vi "ProtocolAnswer.vi"(8 "error in":errorcluster caption="错误输入", 11 "IP":refnum<k5>) -> (0 "error out":errorcluster caption="错误输出", 1 "exit":bool, 3 "IP 2":refnum<k5>)   [LabVIEW 2014]
uses:
  <vilib>/Utility/error.llb/DialogType.ctl
  <vilib>/addons/database/Connection.llb/DB Tools Open Connec (String).vi
  <vilib>/addons/database/_DB Variant To Data/Database Variant To Data.xnode
  <vilib>/addons/database/NI_Database_API.lvlib
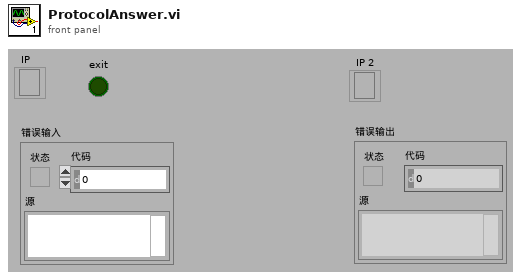
[diagram p1: front panel]
types:
  T1 = enum16{"open", "replace", "create", "open or create", "replace or create", "replace or create with confirmation"}
  T2 = typedef "DialogType.ctl" = u16
  T3 = typedef "NI_Database_API.lvlib/Conn ObjectReference.ctl" = refnum<k1>
  T4 = cluster{string, string, u8, string, u32, string}[]
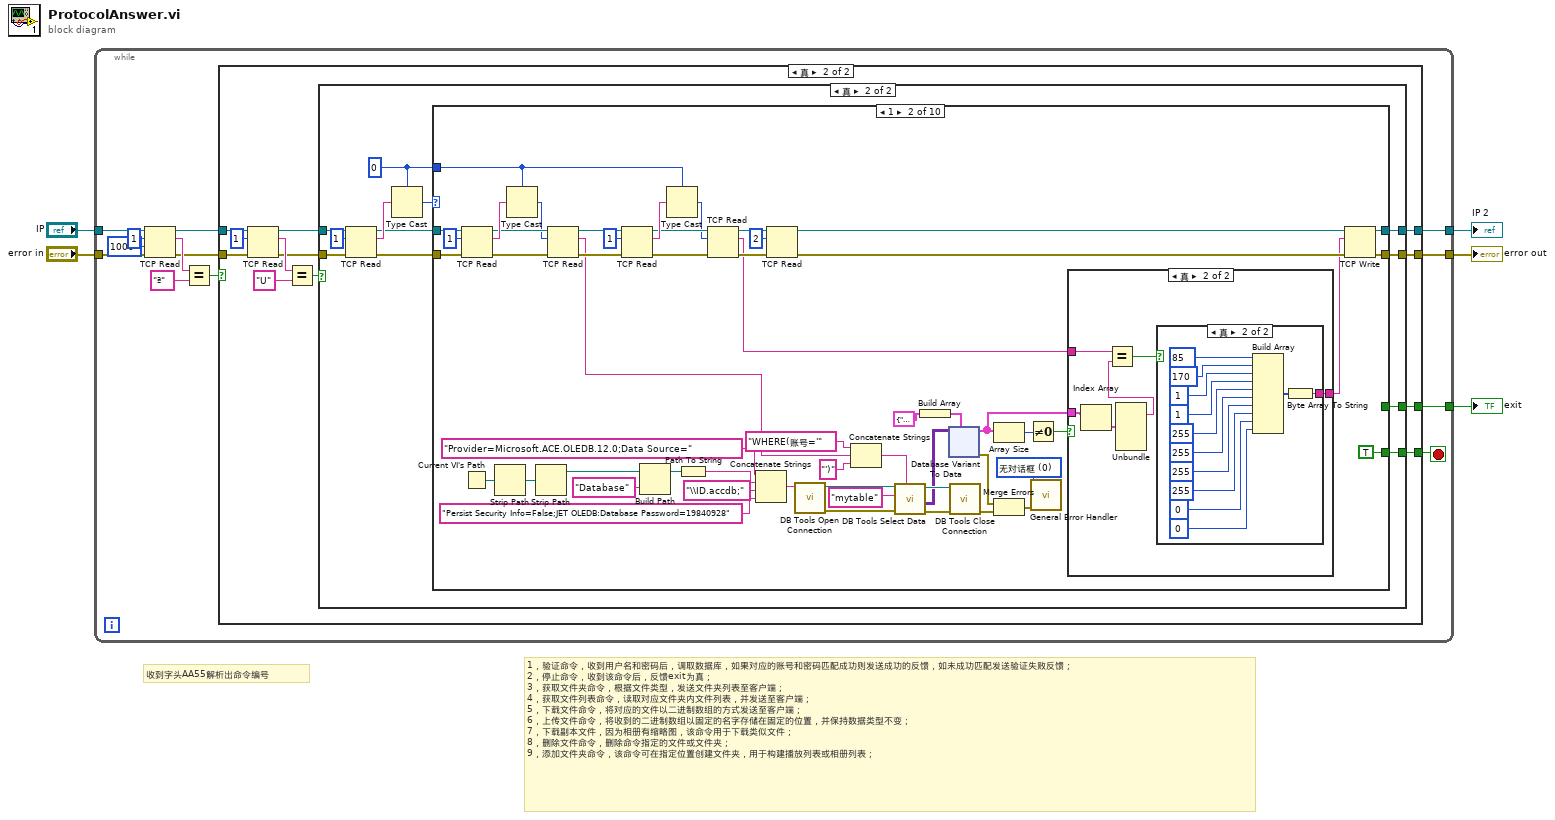
[diagram p0: block diagram]
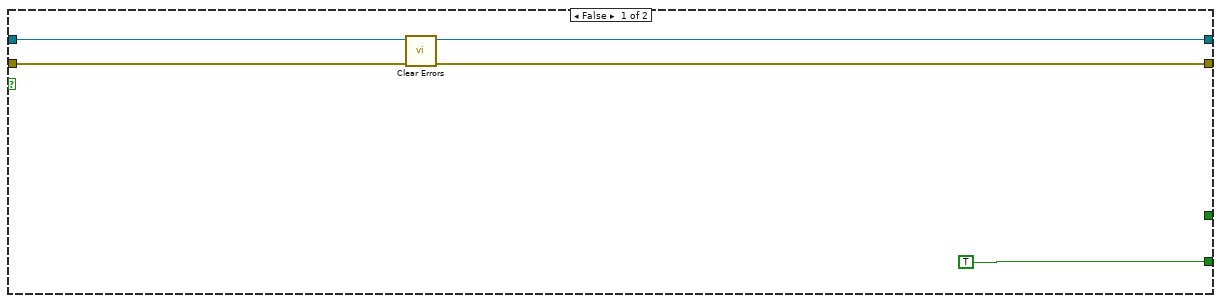
[diagram p2: hidden frame]
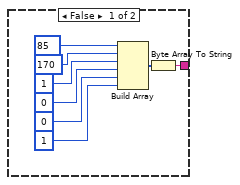
[diagram p5: hidden frame]
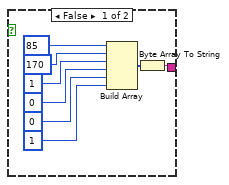
[diagram p6: hidden frame]
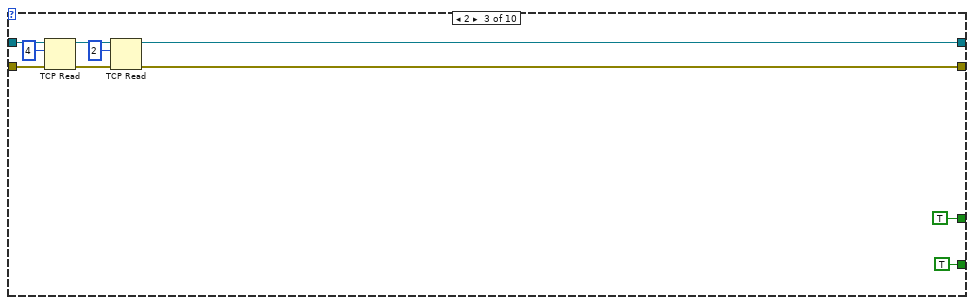
[diagram p7: hidden frame]
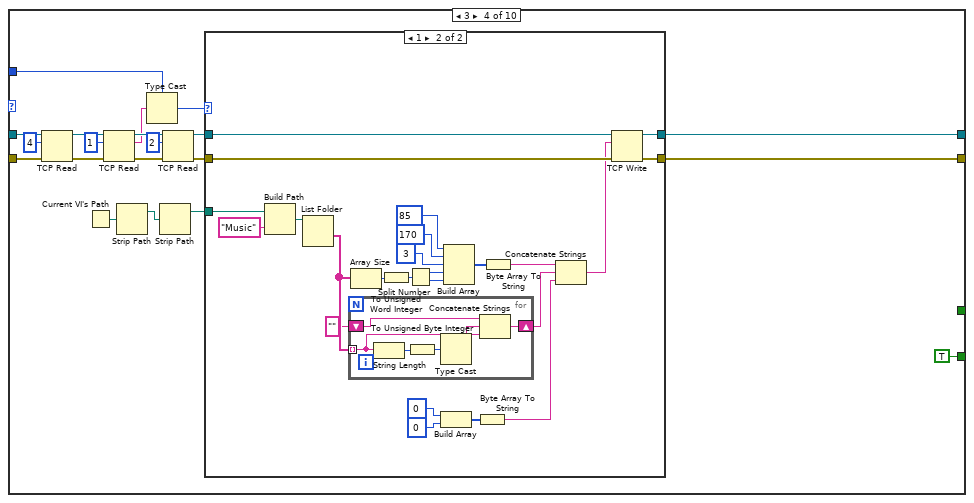
[diagram p8: hidden frame]
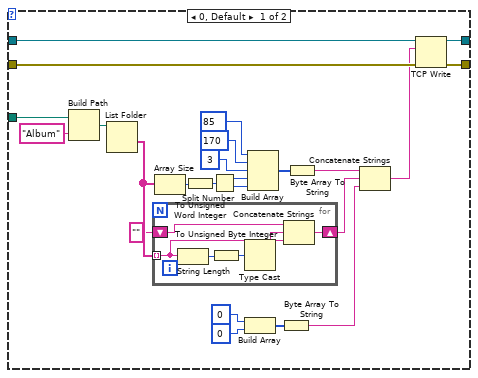
[diagram p9: hidden frame]
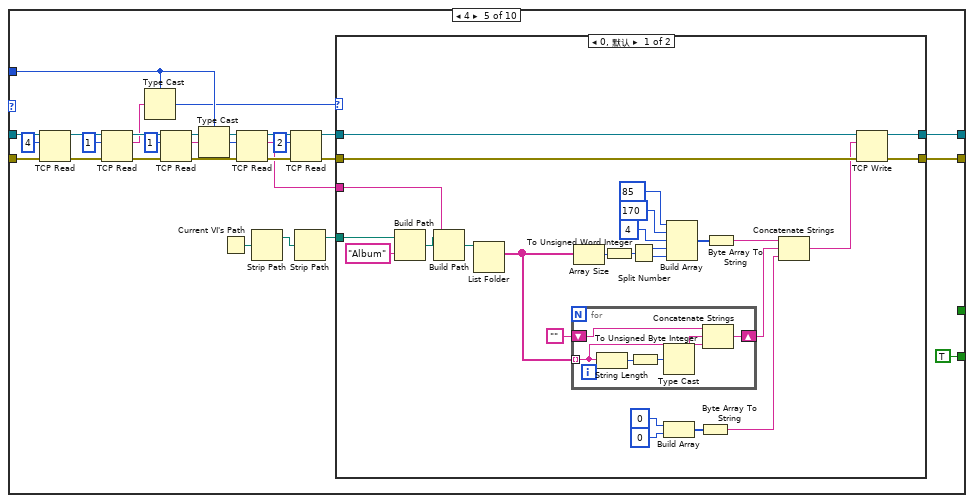
[diagram p10: hidden frame]
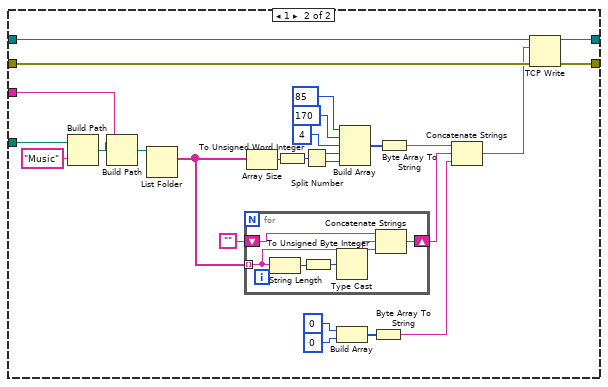
[diagram p11: hidden frame]
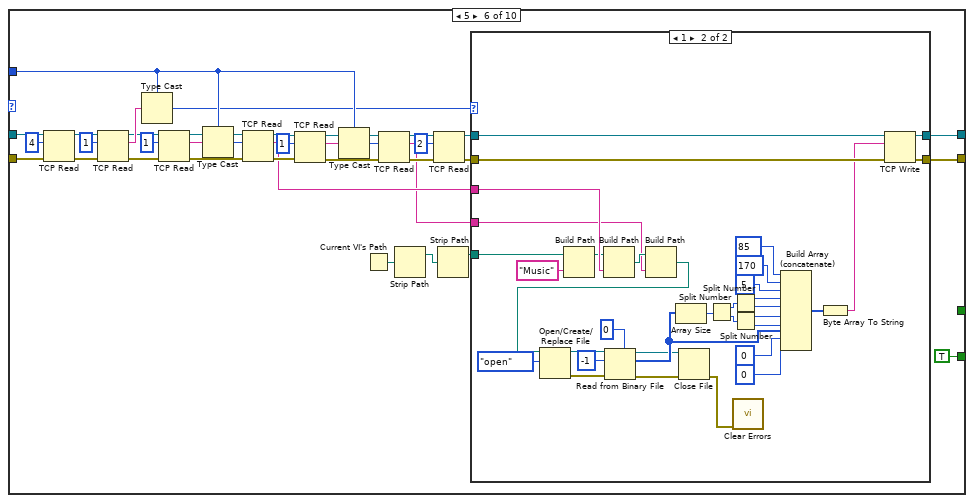
[diagram p12: hidden frame]
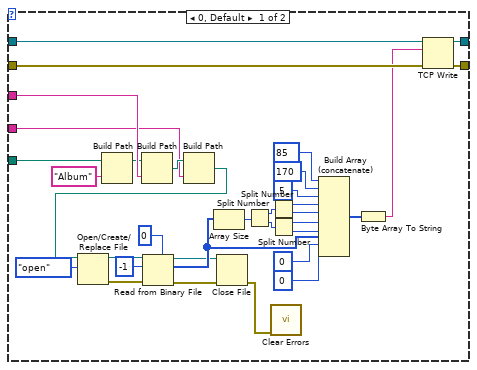
[diagram p13: hidden frame]
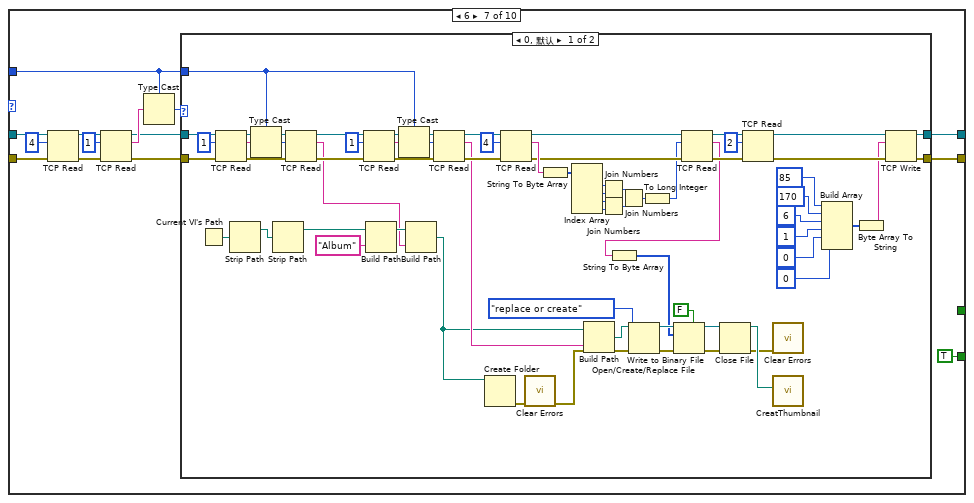
[diagram p14: hidden frame]
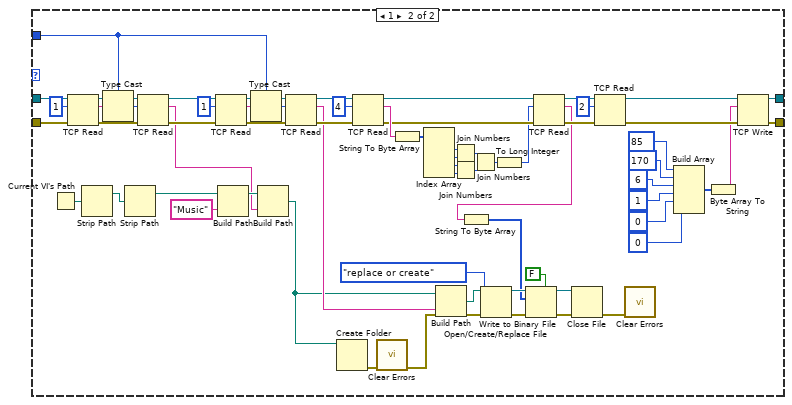
[diagram p15: hidden frame]
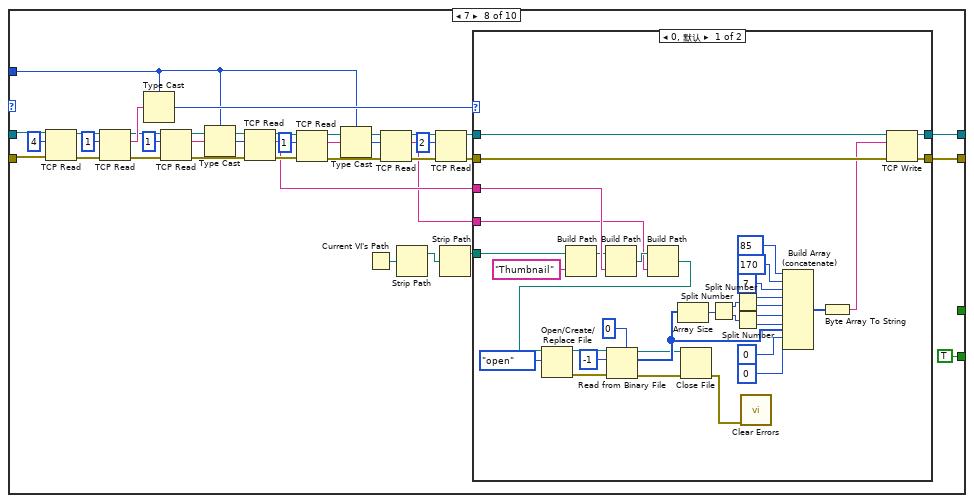
[diagram p16: hidden frame]
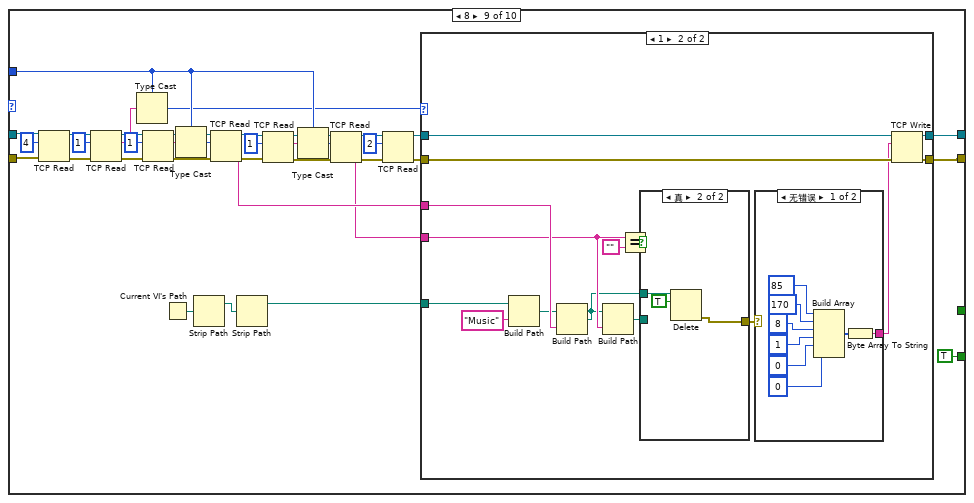
[diagram p18: hidden frame]
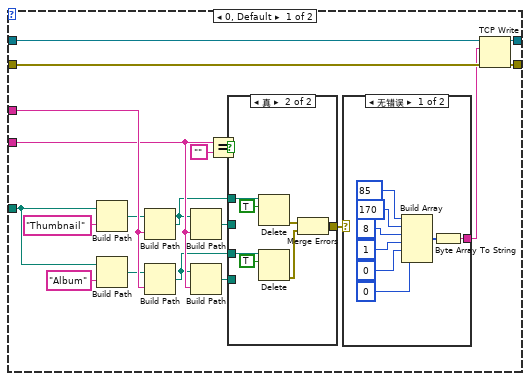
[diagram p19: hidden frame]
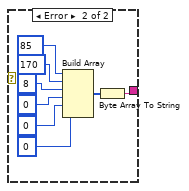
[diagram p20: hidden frame]
diagram:
  # "1，验证命令，收到用户名和密码后，调取数据库，如果对应的账号和密码匹配成功则发送成功的反馈，如未成功匹配发送验证失败反馈；\n2，停止命令，收到该命令后，反馈exit为真；\n3，获取文件夹命令，根据文件类型，发送文件夹列表至客户端；\n4，获取文件列表命令，读取对应文件夹内文件列表，并发送至客户端；\n5，下载文件命令，将对应的文件以二进制数组的方式发送至客户端；\n6，上传文件命令，将收到的二进制数组以固定的名字存储在固定的位置，并保持数据类型不变；\n7，下载副本文件，因为相册有缩略图，该命令用于下载类似文件；\n8，删除文件命令，删除命令指定的文件或文件夹；\n9，添加文件夹命令，该命令可在指定位置创建文件夹，用于构建播放列表或相册列表；"
  # "收到字头AA55解析出命令编号"
  n1 = while {
    tunnel: "IP" -> [w18]
    tunnel: "error in" -> [w17]
    tunnel: [w8] -> w3
    tunnel: [w7] -> w2
    tunnel: [w6] -> w1
    stop <- w9 stop-if-true
    n2 = TCP Read(connection ID=w18, bytes to read=1 ("读取的字节"), error in (no error)=w17, 9:1000 ("超时毫秒(25000)")) -> (connection ID out=w12:refnum<k5>, data out=w13:string, error out=w11:errorcluster)  [unwired: 1 in]
    n3 = Equal?(x=w13, y="ª") -> (x = y?=w10:bool)
    n4 = case shown="真" w10 {
      tunnel: w12 -> [w21 w33]
      tunnel: w11 -> [w20 w32]
      tunnel: [TRUE w26] -> w9
      tunnel: [w21 w25] -> w8
      tunnel: [w19 w24] -> w7
      tunnel: [_ w23] -> w6
      frame False {
        n5 = call <vilib>:"Clear Errors.vi"("error in (no error)"=w20) -> ("error out"=w19:errorcluster)  [unwired: 5 in, 1 out]
      }
      frame True {
        n6 = TCP Read(connection ID=w33, bytes to read=1 ("读取的字节"), error in (no error)=w32) -> (connection ID out=w28:refnum<k5>, data out=w31:string, error out=w27:errorcluster)  [unwired: 2 in]
        n7 = Equal?(x=w31, y="U") -> (x = y?=w29:bool)
        n8 = case shown="真" w29 {
          tunnel: w28 -> [w36 w48]
          tunnel: w27 -> [w35 w47]
          tunnel: [_ w41] -> w26
          tunnel: [w36 w39] -> w25
          tunnel: [w35 w38] -> w24
          tunnel: [_ w37] -> w23
          frame False {
          }
          frame True {
            w40 = u8 0
            n9 = TCP Read(connection ID=w48, bytes to read=1 ("读取的字节"), error in (no error)=w47) -> (connection ID out=w43:refnum<k5>, data out=w45:string, error out=w42:errorcluster)  [unwired: 2 in]
            n10 = Type Cast(type=w40, x=w45) -> (*(type *) &x=w44:u8)
            n11 = case shown="1" w44 {
              tunnel: w43 -> [w50 w102 w343 w363 w444 w551 w633 w770 w851 w970]
              tunnel: w42 -> [w49 w103 w340 w360 w443 w548 w631 w769 w850 w969]
              tunnel: [_ TRUE TRUE TRUE TRUE TRUE TRUE TRUE TRUE TRUE] -> w41
              tunnel: w40 -> [_ w89 _ w355 w440 w542 w621 w771 w849 w968]
              tunnel: [w50 w83 w339 w346 w426 w523 w622 w768 w845 w964] -> w39
              tunnel: [w49 w82 w336 w345 w425 w522 w623 w767 w844 w963] -> w38
              tunnel: [_ _ TRUE _ _ _ _ _ _ _] -> w37
              frame 0, Default {
              }
              frame 1 {
                w52 = T2 0 items=["无对话框", "确定信息", "继续或停止信息", "确定信息＋警告", "继续/停止+警告"] ("type of dialog (OK msg:1)")
                n12 = TCP Read(connection ID=w102, bytes to read=1 ("读取的字节"), error in (no error)=w103) -> (connection ID out=w99:refnum<k5>, data out=w100:string, error out=w98:errorcluster)  [unwired: 2 in]
                n13 = Current VI's Path() -> (path=w79:path)
                n14 = Strip Path(path=w79) -> (stripped path=w80:path)  [unwired: 1 out]
                n15 = Type Cast(type=w89, x=w100) -> (*(type *) &x=w97:u8)
                n16 = Strip Path(path=w80) -> (stripped path=w72:path)  [unwired: 1 out]
                n17 = TCP Read(connection ID=w99, bytes to read=w97, error in (no error)=w98) -> (connection ID out=w91:refnum<k5>, data out=w55:string, error out=w90:errorcluster)  [unwired: 2 in]
                n18 = TCP Read(connection ID=w91, bytes to read=1 ("读取的字节"), error in (no error)=w90) -> (connection ID out=w94:refnum<k5>, data out=w95:string, error out=w93:errorcluster)  [unwired: 2 in]
                n19 = Build Path(base path=w72, name or relative path="Database" ("名称或相对路径")) -> (appended path=w73:path)
                n20 = Type Cast(type=w89, x=w95) -> (*(type *) &x=w92:u8)
                n21 = Path To String(path=w73) -> (string=w63:string)
                n22 = TCP Read(connection ID=w94, bytes to read=w92, error in (no error)=w93) -> (connection ID out=w88:refnum<k5>, data out=w51:string, error out=w87:errorcluster)  [unwired: 2 in]
                n23 = Concatenate Strings("Provider=Microsoft.ACE.OLEDB.12.0;Data Source=", w63, "\\ID.accdb;", "Persist Security Info=False;JET OLEDB:Database Password=19840928" ("字符串")) -> (w65:string)
                n24 = TCP Read(connection ID=w88, bytes to read=2 ("读取的字节"), error in (no error)=w87) -> (connection ID out=w85:refnum<k5>, error out=w84:errorcluster)  [unwired: 2 in, 1 out]
                n25 = call-poly <vilib>:"DB Tools Open Connection.vi"("connection information"=w65) -> ("error out"=w67:errorcluster, "connection reference"=w66:T3)  [unwired: 7 in]
                n26 = Concatenate Strings("WHERE(账号='" ("condition"), w55, "')") -> (w77:string)
                n27 = call <vilib>:"DB Tools Select Data.vi"("condition"=w77, "error in (no error)"=w67, "table"="mytable", "connection reference"=w66) -> ("error out"=w70:errorcluster, "data"=w60:variant[][], "connection reference out"=w69:T3)  [unwired: 2 in]
                n28 = Build Array(cluster{string, string, u8, string, u32, string} {"", "", 0, "", 0, ""}) -> (w58:T4)
                n29 = xnode "Database Variant To Data"("database variant"=w60, "type"=w58) -> ("data"=w53:T4, "error out"=w56:errorcluster)  [unwired: 1 in]
                n30 = call <vilib>:"DB Tools Close Connection.vi"("error in (no error)"=w70, "connection reference"=w69) -> ("error out"=w61:errorcluster)  [unwired: 5 in]
                n31 = Array Size(array=w53) -> (size(s)=w78:i32)
                n32 = Merge Errors(w56, w61) -> (w57:errorcluster)
                n33 = Not Equal To 0?(x=w78) -> (x != 0?=w54:bool)
                n34 = call <vilib>:"General Error Handler.vi"("type of dialog (OK msg:1)"=w52, "error in (no error)"=w57) -> ()  [unwired: 9 in, 5 out]
                n35 = case shown="真" w54 {
                  tunnel: [w105 w118] -> w81
                  tunnel: w53 -> [_ w116]
                  tunnel: w51 -> [_ w115]
                  frame False {
                    n36 = Build Array(u8 85, u8 170, u8 1, u8 0, u8 0, u8 1) -> (w106:u8[])
                    n37 = Byte Array To String(unsigned byte array=w106) -> (string=w105:string)
                  }
                  frame True {
                    n38 = Index Array(array=w116) -> (element=w117:cluster{string, string, u8, string, u32, string})  [unwired: 1 in]
                    n39 = Unbundle(w117) -> (w114:string)  [unwired: 5 out]
                    n40 = Equal?(x=w115, y=w114) -> (x = y?=w113:bool)
                    n41 = case shown="真" w113 {
                      tunnel: [w119 w127] -> w118
                      frame False {
                        n42 = Build Array(u8 85, u8 170, u8 1, u8 0, u8 0, u8 1) -> (w120:u8[])
                        n43 = Byte Array To String(unsigned byte array=w120) -> (string=w119:string)
                      }
                      frame True {
                        n44 = Build Array(u8 85, u8 170, u8 1, u8 1, u8 255, u8 255, u8 255, u8 255, u8 0, u8 0) -> (w128:u8[])
                        n45 = Byte Array To String(unsigned byte array=w128) -> (string=w127:string)
                      }
                    }
                  }
                }
                n46 = TCP Write(connection ID=w85, data in=w81, error in (no error)=w84) -> (connection ID out=w83:refnum<k5>, error out=w82:errorcluster)  [unwired: 1 in, 1 out]
              }
              frame 2 {
                n47 = TCP Read(connection ID=w343, bytes to read=4 ("读取的字节"), error in (no error)=w340) -> (connection ID out=w342:refnum<k5>, error out=w337:errorcluster)  [unwired: 2 in, 1 out]
                n48 = TCP Read(connection ID=w342, bytes to read=2 ("读取的字节"), error in (no error)=w337) -> (connection ID out=w339:refnum<k5>, error out=w336:errorcluster)  [unwired: 2 in, 1 out]
              }
              frame 3 {
                n49 = TCP Read(connection ID=w363, bytes to read=4 ("读取的字节"), error in (no error)=w360) -> (connection ID out=w362:refnum<k5>, error out=w357:errorcluster)  [unwired: 2 in, 1 out]
                n50 = Current VI's Path() -> (path=w351:path)
                n51 = TCP Read(connection ID=w362, bytes to read=1 ("读取的字节"), error in (no error)=w357) -> (connection ID out=w359:refnum<k5>, data out=w356:string, error out=w354:errorcluster)  [unwired: 2 in]
                n52 = Strip Path(path=w351) -> (stripped path=w350:path)  [unwired: 1 out]
                n53 = Type Cast(type=w355, x=w356) -> (*(type *) &x=w352:u8)
                n54 = Strip Path(path=w350) -> (stripped path=w349:path)  [unwired: 1 out]
                n55 = TCP Read(connection ID=w359, bytes to read=2 ("读取的字节"), error in (no error)=w354) -> (connection ID out=w348:refnum<k5>, error out=w347:errorcluster)  [unwired: 2 in, 1 out]
                n56 = case shown="1" w352 {
                  tunnel: w349 -> [w388 w418]
                  tunnel: w348 -> [w376 w406]
                  tunnel: w347 -> [w374 w404]
                  tunnel: [w375 w405] -> w346
                  tunnel: [w373 w403] -> w345
                  frame 0, Default {
                    n57 = Build Path(base path=w388, name or relative path="Album" ("名称或相对路径")) -> (appended path=w386:path)
                    n58 = List Folder(path=w386) -> (folder names=w383:string[])  [unwired: 3 in, 3 out]
                    n59 = for {
                      tunnel: w383 -> [w390] mode=indexing
                      shift-right: [w392] -> w367
                      shift-left: "" -> [w389]
                      n60 = String Length(string=w390) -> (length=w394:i32)
                      n61 = To Unsigned Byte Integer(number=w394) -> (unsigned 8bit integer=w393:u8)
                      n62 = Type Cast(x=w393) -> (*(type *) &x=w391:string)  [unwired: 1 in]
                      n63 = Concatenate Strings(w389, w391, w390) -> (w392:string)
                    }
                    n64 = Array Size(array=w383) -> (size(s)=w385:i32)
                    n65 = To Unsigned Word Integer(number=w385) -> (unsigned 16bit integer=w384:u16)
                    n66 = Split Number(x=w384) -> (hi(x)=w381:u8, lo(x)=w380:u8)
                    n67 = Build Array(u8 0, u8 0) -> (w369:u8[])
                    n68 = Build Array(u8 85, u8 170, u8 3, w381, w380) -> (w372:u8[])
                    n69 = Byte Array To String(unsigned byte array=w369) -> (string=w366:string)
                    n70 = Byte Array To String(unsigned byte array=w372) -> (string=w368:string)
                    n71 = Concatenate Strings(w368, w367, w366) -> (w365:string)
                    n72 = TCP Write(connection ID=w376, data in=w365, error in (no error)=w374) -> (connection ID out=w375:refnum<k5>, error out=w373:errorcluster)  [unwired: 1 in, 1 out]
                  }
                  frame 1 {
                    n73 = Build Path(base path=w418, name or relative path="Music" ("名称或相对路径")) -> (appended path=w416:path)
                    n74 = List Folder(path=w416) -> (folder names=w413:string[])  [unwired: 3 in, 3 out]
                    n75 = for {
                      tunnel: w413 -> [w420] mode=indexing
                      shift-right: [w422] -> w397
                      shift-left: "" -> [w419]
                      n76 = String Length(string=w420) -> (length=w424:i32)
                      n77 = To Unsigned Byte Integer(number=w424) -> (unsigned 8bit integer=w423:u8)
                      n78 = Type Cast(x=w423) -> (*(type *) &x=w421:string)  [unwired: 1 in]
                      n79 = Concatenate Strings(w419, w421, w420) -> (w422:string)
                    }
                    n80 = Array Size(array=w413) -> (size(s)=w415:i32)
                    n81 = To Unsigned Word Integer(number=w415) -> (unsigned 16bit integer=w414:u16)
                    n82 = Split Number(x=w414) -> (hi(x)=w411:u8, lo(x)=w410:u8)
                    n83 = Build Array(u8 0, u8 0) -> (w399:u8[])
                    n84 = Build Array(u8 85, u8 170, u8 3, w411, w410) -> (w402:u8[])
                    n85 = Byte Array To String(unsigned byte array=w399) -> (string=w396:string)
                    n86 = Byte Array To String(unsigned byte array=w402) -> (string=w398:string)
                    n87 = Concatenate Strings(w398, w397, w396) -> (w395:string)
                    n88 = TCP Write(connection ID=w406, data in=w395, error in (no error)=w404) -> (connection ID out=w405:refnum<k5>, error out=w403:errorcluster)  [unwired: 1 in, 1 out]
                  }
                }
              }
              frame 4 {
                n89 = TCP Read(connection ID=w444, bytes to read=4 ("读取的字节"), error in (no error)=w443) -> (connection ID out=w451:refnum<k5>, error out=w447:errorcluster)  [unwired: 2 in, 1 out]
                n90 = TCP Read(connection ID=w451, bytes to read=1 ("读取的字节"), error in (no error)=w447) -> (connection ID out=w449:refnum<k5>, data out=w442:string, error out=w446:errorcluster)  [unwired: 2 in]
                n91 = Type Cast(type=w440, x=w442) -> (*(type *) &x=w433:u8)
                n92 = TCP Read(connection ID=w449, bytes to read=1 ("读取的字节"), error in (no error)=w446) -> (connection ID out=w439:refnum<k5>, data out=w441:string, error out=w438:errorcluster)  [unwired: 2 in]
                n93 = Type Cast(type=w440, x=w441) -> (*(type *) &x=w437:u8)
                n94 = Current VI's Path() -> (path=w429:path)
                n95 = TCP Read(connection ID=w439, bytes to read=w437, error in (no error)=w438) -> (connection ID out=w436:refnum<k5>, data out=w430:string, error out=w435:errorcluster)  [unwired: 2 in]
                n96 = Strip Path(path=w429) -> (stripped path=w428:path)  [unwired: 1 out]
                n97 = TCP Read(connection ID=w436, bytes to read=2 ("读取的字节"), error in (no error)=w435) -> (connection ID out=w432:refnum<k5>, error out=w431:errorcluster)  [unwired: 2 in, 1 out]
                n98 = Strip Path(path=w428) -> (stripped path=w427:path)  [unwired: 1 out]
                n99 = case shown="0, 默认" w433 {
                  tunnel: w432 -> [w474 w506]
                  tunnel: w431 -> [w456 w488]
                  tunnel: w430 -> [w475 w507]
                  tunnel: w427 -> [w477 w509]
                  tunnel: [w457 w489] -> w426
                  tunnel: [w455 w487] -> w425
                  frame 0, Default {
                    n100 = Build Path(base path=w477, name or relative path="Album" ("名称或相对路径")) -> (appended path=w476:path)
                    n101 = Build Path(base path=w476, name or relative path=w475) -> (appended path=w473:path)
                    n102 = List Folder(path=w473) -> (filenames=w453:string[])  [unwired: 3 in, 3 out]
                    n103 = for {
                      tunnel: w453 -> [w480] mode=indexing
                      shift-right: [w482] -> w471
                      shift-left: "" -> [w479]
                      n104 = String Length(string=w480) -> (length=w484:i32)
                      n105 = To Unsigned Byte Integer(number=w484) -> (unsigned 8bit integer=w483:u8)
                      n106 = Type Cast(x=w483) -> (*(type *) &x=w481:string)  [unwired: 1 in]
                      n107 = Concatenate Strings(w479, w481, w480) -> (w482:string)
                    }
                    n108 = Array Size(array=w453) -> (size(s)=w458:i32)
                    n109 = To Unsigned Word Integer(number=w458) -> (unsigned 16bit integer=w459:u16)
                    n110 = Split Number(x=w459) -> (hi(x)=w461:u8, lo(x)=w462:u8)
                    n111 = Build Array(u8 0, u8 0) -> (w469:u8[])
                    n112 = Build Array(u8 85, u8 170, u8 4, w461, w462) -> (w466:u8[])
                    n113 = Byte Array To String(unsigned byte array=w469) -> (string=w472:string)
                    n114 = Byte Array To String(unsigned byte array=w466) -> (string=w470:string)
                    n115 = Concatenate Strings(w470, w471, w472) -> (w454:string)
                    n116 = TCP Write(connection ID=w474, data in=w454, error in (no error)=w456) -> (connection ID out=w457:refnum<k5>, error out=w455:errorcluster)  [unwired: 1 in, 1 out]
                  }
                  frame 1 {
                    n117 = Build Path(base path=w509, name or relative path="Music" ("名称或相对路径")) -> (appended path=w508:path)
                    n118 = Build Path(base path=w508, name or relative path=w507) -> (appended path=w505:path)
                    n119 = List Folder(path=w505) -> (filenames=w485:string[])  [unwired: 3 in, 3 out]
                    n120 = for {
                      tunnel: w485 -> [w512] mode=indexing
                      shift-right: [w514] -> w503
                      shift-left: "" -> [w511]
                      n121 = String Length(string=w512) -> (length=w516:i32)
                      n122 = To Unsigned Byte Integer(number=w516) -> (unsigned 8bit integer=w515:u8)
                      n123 = Type Cast(x=w515) -> (*(type *) &x=w513:string)  [unwired: 1 in]
                      n124 = Concatenate Strings(w511, w513, w512) -> (w514:string)
                    }
                    n125 = Array Size(array=w485) -> (size(s)=w490:i32)
                    n126 = To Unsigned Word Integer(number=w490) -> (unsigned 16bit integer=w491:u16)
                    n127 = Split Number(x=w491) -> (hi(x)=w493:u8, lo(x)=w494:u8)
                    n128 = Build Array(u8 0, u8 0) -> (w501:u8[])
                    n129 = Build Array(u8 85, u8 170, u8 4, w493, w494) -> (w498:u8[])
                    n130 = Byte Array To String(unsigned byte array=w501) -> (string=w504:string)
                    n131 = Byte Array To String(unsigned byte array=w498) -> (string=w502:string)
                    n132 = Concatenate Strings(w502, w503, w504) -> (w486:string)
                    n133 = TCP Write(connection ID=w506, data in=w486, error in (no error)=w488) -> (connection ID out=w489:refnum<k5>, error out=w487:errorcluster)  [unwired: 1 in, 1 out]
                  }
                }
              }
              frame 5 {
                n134 = TCP Read(connection ID=w551, bytes to read=4 ("读取的字节"), error in (no error)=w548) -> (connection ID out=w550:refnum<k5>, error out=w547:errorcluster)  [unwired: 2 in, 1 out]
                n135 = TCP Read(connection ID=w550, bytes to read=1 ("读取的字节"), error in (no error)=w547) -> (connection ID out=w544:refnum<k5>, data out=w545:string, error out=w543:errorcluster)  [unwired: 2 in]
                n136 = Type Cast(type=w542, x=w545) -> (*(type *) &x=w524:u8)
                n137 = TCP Read(connection ID=w544, bytes to read=1 ("读取的字节"), error in (no error)=w543) -> (connection ID out=w538:refnum<k5>, data out=w521:string, error out=w537:errorcluster)  [unwired: 2 in]
                n138 = Type Cast(type=w542, x=w521) -> (*(type *) &x=w536:u8)
                n139 = TCP Read(connection ID=w538, bytes to read=w536, error in (no error)=w537) -> (connection ID out=w531:refnum<k5>, data out=w518:string, error out=w530:errorcluster)  [unwired: 2 in]
                n140 = TCP Read(connection ID=w531, bytes to read=1 ("读取的字节"), error in (no error)=w530) -> (connection ID out=w534:refnum<k5>, data out=w520:string, error out=w533:errorcluster)  [unwired: 2 in]
                n141 = Type Cast(type=w542, x=w520) -> (*(type *) &x=w532:u8)
                n142 = Current VI's Path() -> (path=w541:path)
                n143 = TCP Read(connection ID=w534, bytes to read=w532, error in (no error)=w533) -> (connection ID out=w528:refnum<k5>, data out=w517:string, error out=w529:errorcluster)  [unwired: 2 in]
                n144 = Strip Path(path=w541) -> (stripped path=w540:path)  [unwired: 1 out]
                n145 = TCP Read(connection ID=w528, bytes to read=2 ("读取的字节"), error in (no error)=w529) -> (connection ID out=w526:refnum<k5>, error out=w525:errorcluster)  [unwired: 2 in, 1 out]
                n146 = Strip Path(path=w540) -> (stripped path=w519:path)  [unwired: 1 out]
                n147 = case shown="1" w524 {
                  tunnel: w526 -> [w582 w616]
                  tunnel: w525 -> [w562 w596]
                  tunnel: [w563 w597] -> w523
                  tunnel: [w561 w595] -> w522
                  tunnel: w518 -> [w585 w619]
                  tunnel: w517 -> [w583 w617]
                  tunnel: w519 -> [w586 w620]
                  frame 0, Default {
                    n148 = Build Path(base path=w586, name or relative path="Album" ("名称或相对路径")) -> (appended path=w581:path)
                    n149 = Build Path(base path=w581, name or relative path=w585) -> (appended path=w584:path)
                    n150 = Build Path(base path=w584, name or relative path=w583) -> (appended path=w564:path)
                    n151 = Open/Create/Replace File(file path (use dialog)=w564, operation (0:open)=T1."open" ("操作(0:open)")) -> (refnum out=w567:refnum<file>, error out=w570:errorcluster)  [unwired: 4 in, 1 out]
                    n152 = Read from Binary File(5:u8 0, 8:w570, 10:-1 ("总数(1)"), 11:w567) -> (0:w568:errorcluster, 2:w575:u8[], 3:w569:refnum<file>)  [unwired: 2 in, 1 out]
                    n153 = Array Size(array=w575) -> (size(s)=w571:i32)
                    n154 = Close File(refnum=w569, error in=w568) -> (error out=w553:errorcluster)  [unwired: 1 out]
                    n155 = Split Number(x=w571) -> (hi(x)=w572:u16, lo(x)=w573:u16)
                    n156 = Split Number(x=w572) -> (hi(x)=w574:u8, lo(x)=w576:u8)
                    n157 = Split Number(x=w573) -> (hi(x)=w577:u8, lo(x)=w578:u8)
                    n158 = call <vilib>:"Clear Errors.vi"("error in (no error)"=w553) -> ()  [unwired: 5 in, 2 out]
                    n159 = Build Array (concatenate)(u8 85, u8 170, u8 5, w574, w576, w577, w578, w575, u8 0, u8 0) -> (w579:u8[])
                    n160 = Byte Array To String(unsigned byte array=w579) -> (string=w555:string)
                    n161 = TCP Write(connection ID=w582, data in=w555, error in (no error)=w562) -> (connection ID out=w563:refnum<k5>, error out=w561:errorcluster)  [unwired: 1 in, 1 out]
                  }
                  frame 1 {
                    n162 = Build Path(base path=w620, name or relative path="Music" ("名称或相对路径")) -> (appended path=w615:path)
                    n163 = Build Path(base path=w615, name or relative path=w619) -> (appended path=w618:path)
                    n164 = Build Path(base path=w618, name or relative path=w617) -> (appended path=w598:path)
                    n165 = Open/Create/Replace File(file path (use dialog)=w598, operation (0:open)=T1."open" ("操作(0:open)")) -> (refnum out=w601:refnum<file>, error out=w604:errorcluster)  [unwired: 4 in, 1 out]
                    n166 = Read from Binary File(5:u8 0, 8:w604, 10:-1 ("总数(1)"), 11:w601) -> (0:w602:errorcluster, 2:w609:u8[], 3:w603:refnum<file>)  [unwired: 2 in, 1 out]
                    n167 = Array Size(array=w609) -> (size(s)=w605:i32)
                    n168 = Close File(refnum=w603, error in=w602) -> (error out=w587:errorcluster)  [unwired: 1 out]
                    n169 = Split Number(x=w605) -> (hi(x)=w606:u16, lo(x)=w607:u16)
                    n170 = Split Number(x=w606) -> (hi(x)=w608:u8, lo(x)=w610:u8)
                    n171 = Split Number(x=w607) -> (hi(x)=w611:u8, lo(x)=w612:u8)
                    n172 = call <vilib>:"Clear Errors.vi"("error in (no error)"=w587) -> ()  [unwired: 5 in, 2 out]
                    n173 = Build Array (concatenate)(u8 85, u8 170, u8 5, w608, w610, w611, w612, w609, u8 0, u8 0) -> (w613:u8[])
                    n174 = Byte Array To String(unsigned byte array=w613) -> (string=w589:string)
                    n175 = TCP Write(connection ID=w616, data in=w589, error in (no error)=w596) -> (connection ID out=w597:refnum<k5>, error out=w595:errorcluster)  [unwired: 1 in, 1 out]
                  }
                }
              }
              frame 6 {
                n176 = TCP Read(connection ID=w633, bytes to read=4 ("读取的字节"), error in (no error)=w631) -> (connection ID out=w632:refnum<k5>, error out=w628:errorcluster)  [unwired: 2 in, 1 out]
                n177 = TCP Read(connection ID=w632, bytes to read=1 ("读取的字节"), error in (no error)=w628) -> (connection ID out=w625:refnum<k5>, data out=w627:string, error out=w624:errorcluster)  [unwired: 2 in]
                n178 = Type Cast(type=w621, x=w627) -> (*(type *) &x=w626:u8)
                n179 = case shown="0, 默认" w626 {
                  tunnel: w625 -> [w687 w752]
                  tunnel: [w660 w725] -> w623
                  tunnel: w624 -> [w688 w753]
                  tunnel: [w657 w722] -> w622
                  tunnel: w621 -> [w686 w751]
                  frame 0, Default {
                    n180 = Current VI's Path() -> (path=w655:path)
                    n181 = TCP Read(connection ID=w687, bytes to read=1 ("读取的字节"), error in (no error)=w688) -> (connection ID out=w699:refnum<k5>, data out=w690:string, error out=w698:errorcluster)  [unwired: 2 in]
                    n182 = Strip Path(path=w655) -> (stripped path=w654:path)  [unwired: 1 out]
                    n183 = Type Cast(type=w686, x=w690) -> (*(type *) &x=w697:u8)
                    n184 = Strip Path(path=w654) -> (stripped path=w651:path)  [unwired: 1 out]
                    n185 = TCP Read(connection ID=w699, bytes to read=w697, error in (no error)=w698) -> (connection ID out=w692:refnum<k5>, data out=w650:string, error out=w691:errorcluster)  [unwired: 2 in]
                    n186 = TCP Read(connection ID=w692, bytes to read=1 ("读取的字节"), error in (no error)=w691) -> (connection ID out=w695:refnum<k5>, data out=w689:string, error out=w694:errorcluster)  [unwired: 2 in]
                    n187 = Build Path(base path=w651, name or relative path="Album" ("名称或相对路径")) -> (appended path=w653:path)
                    n188 = Type Cast(type=w686, x=w689) -> (*(type *) &x=w693:u8)
                    n189 = Build Path(base path=w653, name or relative path=w650) -> (appended path=w637:path)
                    n190 = TCP Read(connection ID=w695, bytes to read=w693, error in (no error)=w694) -> (connection ID out=w684:refnum<k5>, data out=w638:string, error out=w685:errorcluster)  [unwired: 2 in]
                    n191 = Create Folder(path (use dialog)=w637) -> (error out=w647:errorcluster)  [unwired: 2 in, 2 out]
                    n192 = TCP Read(connection ID=w684, bytes to read=4 ("读取的字节"), error in (no error)=w685) -> (connection ID out=w673:refnum<k5>, data out=w682:string, error out=w672:errorcluster)  [unwired: 2 in]
                    n193 = call <vilib>:"Clear Errors.vi"("error in (no error)"=w647) -> ("error out"=w648:errorcluster)  [unwired: 5 in, 1 out]
                    n194 = String To Byte Array(string=w682) -> (unsigned byte array=w681:u8[])
                    n195 = Index Array(array=w681) -> (element #1=w679:u8, element #2=w680:u8, element #3=w677:u8, element #4=w678:u8)  [unwired: 4 in]
                    n196 = Build Path(base path=w637, name or relative path=w638) -> (appended path=w640:path)
                    n197 = Join Numbers(hi=w679, lo=w680) -> ((hi.lo)=w675:u16)
                    n198 = Join Numbers(hi=w677, lo=w678) -> ((hi.lo)=w676:u16)
                    n199 = Join Numbers(hi=w675, lo=w676) -> ((hi.lo)=w674:u32)
                    n200 = Open/Create/Replace File(file path (use dialog)=w640, error in=w648, operation (0:open)=T1."replace or create" ("操作(0:open)")) -> (refnum out=w642:refnum<file>, error out=w643:errorcluster)  [unwired: 3 in, 1 out]
                    n201 = To Long Integer(number=w674) -> (32bit integer=w671:i32)
                    n202 = TCP Read(connection ID=w673, bytes to read=w671, error in (no error)=w672) -> (connection ID out=w669:refnum<k5>, data out=w649:string, error out=w670:errorcluster)  [unwired: 2 in]
                    n203 = String To Byte Array(string=w649) -> (unsigned byte array=w639:u8[])
                    n204 = Write to Binary File(file (use dialog)=w642, data=w639, error in=w643, 5:FALSE ("预置数组或字符串大小？(T)")) -> (refnum out=w645:refnum<file>, error out=w644:errorcluster)  [unwired: 2 in, 1 out]
                    n205 = Close File(refnum=w645, error in=w644) -> (path=w636:path, error out=w635:errorcluster)
                    n206 = TCP Read(connection ID=w669, bytes to read=2 ("读取的字节"), error in (no error)=w670) -> (connection ID out=w658:refnum<k5>, error out=w659:errorcluster)  [unwired: 2 in, 1 out]
                    n207 = call <vilib>:"Clear Errors.vi"("error in (no error)"=w635) -> ()  [unwired: 5 in, 2 out]
                    n208 = call "CreatThumbnail.vi"("file"=w636) -> ()  [unwired: 11 in]
                    n209 = Build Array(u8 85, u8 170, u8 6, u8 1 ("元素"), u8 0, u8 0) -> (w667:u8[])
                    n210 = Byte Array To String(unsigned byte array=w667) -> (string=w656:string)
                    n211 = TCP Write(connection ID=w658, data in=w656, error in (no error)=w659) -> (connection ID out=w657:refnum<k5>, error out=w660:errorcluster)  [unwired: 1 in, 1 out]
                  }
                  frame 1 {
                    n212 = Current VI's Path() -> (path=w720:path)
                    n213 = TCP Read(connection ID=w752, bytes to read=1 ("读取的字节"), error in (no error)=w753) -> (connection ID out=w764:refnum<k5>, data out=w755:string, error out=w763:errorcluster)  [unwired: 2 in]
                    n214 = Strip Path(path=w720) -> (stripped path=w719:path)  [unwired: 1 out]
                    n215 = Type Cast(type=w751, x=w755) -> (*(type *) &x=w762:u8)
                    n216 = Strip Path(path=w719) -> (stripped path=w716:path)  [unwired: 1 out]
                    n217 = TCP Read(connection ID=w764, bytes to read=w762, error in (no error)=w763) -> (connection ID out=w757:refnum<k5>, data out=w715:string, error out=w756:errorcluster)  [unwired: 2 in]
                    n218 = TCP Read(connection ID=w757, bytes to read=1 ("读取的字节"), error in (no error)=w756) -> (connection ID out=w760:refnum<k5>, data out=w754:string, error out=w759:errorcluster)  [unwired: 2 in]
                    n219 = Build Path(base path=w716, name or relative path="Music" ("名称或相对路径")) -> (appended path=w718:path)
                    n220 = Type Cast(type=w751, x=w754) -> (*(type *) &x=w758:u8)
                    n221 = Build Path(base path=w718, name or relative path=w715) -> (appended path=w702:path)
                    n222 = TCP Read(connection ID=w760, bytes to read=w758, error in (no error)=w759) -> (connection ID out=w749:refnum<k5>, data out=w703:string, error out=w750:errorcluster)  [unwired: 2 in]
                    n223 = Create Folder(path (use dialog)=w702) -> (error out=w712:errorcluster)  [unwired: 2 in, 2 out]
                    n224 = TCP Read(connection ID=w749, bytes to read=4 ("读取的字节"), error in (no error)=w750) -> (connection ID out=w738:refnum<k5>, data out=w747:string, error out=w737:errorcluster)  [unwired: 2 in]
                    n225 = call <vilib>:"Clear Errors.vi"("error in (no error)"=w712) -> ("error out"=w713:errorcluster)  [unwired: 5 in, 1 out]
                    n226 = String To Byte Array(string=w747) -> (unsigned byte array=w746:u8[])
                    n227 = Index Array(array=w746) -> (element #1=w744:u8, element #2=w745:u8, element #3=w742:u8, element #4=w743:u8)  [unwired: 4 in]
                    n228 = Build Path(base path=w702, name or relative path=w703) -> (appended path=w705:path)
                    n229 = Join Numbers(hi=w744, lo=w745) -> ((hi.lo)=w740:u16)
                    n230 = Join Numbers(hi=w742, lo=w743) -> ((hi.lo)=w741:u16)
                    n231 = Join Numbers(hi=w740, lo=w741) -> ((hi.lo)=w739:u32)
                    n232 = Open/Create/Replace File(file path (use dialog)=w705, error in=w713, operation (0:open)=T1."replace or create" ("操作(0:open)")) -> (refnum out=w707:refnum<file>, error out=w708:errorcluster)  [unwired: 3 in, 1 out]
                    n233 = To Long Integer(number=w739) -> (32bit integer=w736:i32)
                    n234 = TCP Read(connection ID=w738, bytes to read=w736, error in (no error)=w737) -> (connection ID out=w734:refnum<k5>, data out=w714:string, error out=w735:errorcluster)  [unwired: 2 in]
                    n235 = String To Byte Array(string=w714) -> (unsigned byte array=w704:u8[])
                    n236 = Write to Binary File(file (use dialog)=w707, data=w704, error in=w708, 5:FALSE ("预置数组或字符串大小？(T)")) -> (refnum out=w710:refnum<file>, error out=w709:errorcluster)  [unwired: 2 in, 1 out]
                    n237 = Close File(refnum=w710, error in=w709) -> (error out=w701:errorcluster)  [unwired: 1 out]
                    n238 = TCP Read(connection ID=w734, bytes to read=2 ("读取的字节"), error in (no error)=w735) -> (connection ID out=w723:refnum<k5>, error out=w724:errorcluster)  [unwired: 2 in, 1 out]
                    n239 = call <vilib>:"Clear Errors.vi"("error in (no error)"=w701) -> ()  [unwired: 5 in, 2 out]
                    n240 = Build Array(u8 85, u8 170, u8 6, u8 1 ("元素"), u8 0, u8 0) -> (w732:u8[])
                    n241 = Byte Array To String(unsigned byte array=w732) -> (string=w721:string)
                    n242 = TCP Write(connection ID=w723, data in=w721, error in (no error)=w724) -> (connection ID out=w722:refnum<k5>, error out=w725:errorcluster)  [unwired: 1 in, 1 out]
                  }
                }
              }
              frame 7 {
                n243 = TCP Read(connection ID=w770, bytes to read=4 ("读取的字节"), error in (no error)=w769) -> (connection ID out=w801:refnum<k5>, error out=w799:errorcluster)  [unwired: 2 in, 1 out]
                n244 = TCP Read(connection ID=w801, bytes to read=1 ("读取的字节"), error in (no error)=w799) -> (connection ID out=w796:refnum<k5>, data out=w797:string, error out=w795:errorcluster)  [unwired: 2 in]
                n245 = Type Cast(type=w771, x=w797) -> (*(type *) &x=w777:u8)
                n246 = TCP Read(connection ID=w796, bytes to read=1 ("读取的字节"), error in (no error)=w795) -> (connection ID out=w791:refnum<k5>, data out=w776:string, error out=w790:errorcluster)  [unwired: 2 in]
                n247 = Type Cast(type=w771, x=w776) -> (*(type *) &x=w789:u8)
                n248 = TCP Read(connection ID=w791, bytes to read=w789, error in (no error)=w790) -> (connection ID out=w784:refnum<k5>, data out=w773:string, error out=w783:errorcluster)  [unwired: 2 in]
                n249 = TCP Read(connection ID=w784, bytes to read=1 ("读取的字节"), error in (no error)=w783) -> (connection ID out=w787:refnum<k5>, data out=w775:string, error out=w786:errorcluster)  [unwired: 2 in]
                n250 = Type Cast(type=w771, x=w775) -> (*(type *) &x=w785:u8)
                n251 = Current VI's Path() -> (path=w794:path)
                n252 = TCP Read(connection ID=w787, bytes to read=w785, error in (no error)=w786) -> (connection ID out=w781:refnum<k5>, data out=w772:string, error out=w782:errorcluster)  [unwired: 2 in]
                n253 = Strip Path(path=w794) -> (stripped path=w793:path)  [unwired: 1 out]
                n254 = TCP Read(connection ID=w781, bytes to read=2 ("读取的字节"), error in (no error)=w782) -> (connection ID out=w779:refnum<k5>, error out=w778:errorcluster)  [unwired: 2 in, 1 out]
                n255 = Strip Path(path=w793) -> (stripped path=w774:path)  [unwired: 1 out]
                n256 = case shown="0, 默认" w777 {
                  tunnel: w779 -> [w831 w837]
                  tunnel: w778 -> [w811 w836]
                  tunnel: [w812 w837] -> w768
                  tunnel: [w810 w836] -> w767
                  tunnel: w773 -> [w834 _]
                  tunnel: w772 -> [w832 _]
                  tunnel: w774 -> [w835 _]
                  frame 0, Default {
                    n257 = Build Path(base path=w835, name or relative path="Thumbnail" ("名称或相对路径")) -> (appended path=w830:path)
                    n258 = Build Path(base path=w830, name or relative path=w834) -> (appended path=w833:path)
                    n259 = Build Path(base path=w833, name or relative path=w832) -> (appended path=w813:path)
                    n260 = Open/Create/Replace File(file path (use dialog)=w813, operation (0:open)=T1."open" ("操作(0:open)")) -> (refnum out=w816:refnum<file>, error out=w819:errorcluster)  [unwired: 4 in, 1 out]
                    n261 = Read from Binary File(5:u8 0, 8:w819, 10:-1 ("总数(1)"), 11:w816) -> (0:w817:errorcluster, 2:w824:u8[], 3:w818:refnum<file>)  [unwired: 2 in, 1 out]
                    n262 = Array Size(array=w824) -> (size(s)=w820:i32)
                    n263 = Close File(refnum=w818, error in=w817) -> (error out=w802:errorcluster)  [unwired: 1 out]
                    n264 = Split Number(x=w820) -> (hi(x)=w821:u16, lo(x)=w822:u16)
                    n265 = Split Number(x=w821) -> (hi(x)=w823:u8, lo(x)=w825:u8)
                    n266 = Split Number(x=w822) -> (hi(x)=w826:u8, lo(x)=w827:u8)
                    n267 = call <vilib>:"Clear Errors.vi"("error in (no error)"=w802) -> ()  [unwired: 5 in, 2 out]
                    n268 = Build Array (concatenate)(u8 85, u8 170, u8 7, w823, w825, w826, w827, w824, u8 0, u8 0) -> (w828:u8[])
                    n269 = Byte Array To String(unsigned byte array=w828) -> (string=w804:string)
                    n270 = TCP Write(connection ID=w831, data in=w804, error in (no error)=w811) -> (connection ID out=w812:refnum<k5>, error out=w810:errorcluster)  [unwired: 1 in, 1 out]
                  }
                  frame 1 {
                  }
                }
              }
              frame 8 {
                n271 = TCP Read(connection ID=w851, bytes to read=4 ("读取的字节"), error in (no error)=w850) -> (connection ID out=w872:refnum<k5>, error out=w870:errorcluster)  [unwired: 2 in, 1 out]
                n272 = TCP Read(connection ID=w872, bytes to read=1 ("读取的字节"), error in (no error)=w870) -> (connection ID out=w867:refnum<k5>, data out=w868:string, error out=w866:errorcluster)  [unwired: 2 in]
                n273 = Type Cast(type=w849, x=w868) -> (*(type *) &x=w848:u8)
                n274 = TCP Read(connection ID=w867, bytes to read=1 ("读取的字节"), error in (no error)=w866) -> (connection ID out=w864:refnum<k5>, data out=w852:string, error out=w863:errorcluster)  [unwired: 2 in]
                n275 = Current VI's Path() -> (path=w840:path)
                n276 = Type Cast(type=w849, x=w852) -> (*(type *) &x=w862:u8)
                n277 = Strip Path(path=w840) -> (stripped path=w839:path)  [unwired: 1 out]
                n278 = TCP Read(connection ID=w864, bytes to read=w862, error in (no error)=w863) -> (connection ID out=w857:refnum<k5>, data out=w842:string, error out=w856:errorcluster)  [unwired: 2 in]
                n279 = Strip Path(path=w839) -> (stripped path=w838:path)  [unwired: 1 out]
                n280 = TCP Read(connection ID=w857, bytes to read=1 ("读取的字节"), error in (no error)=w856) -> (connection ID out=w860:refnum<k5>, data out=w843:string, error out=w859:errorcluster)  [unwired: 2 in]
                n281 = Type Cast(type=w849, x=w843) -> (*(type *) &x=w858:u8)
                n282 = TCP Read(connection ID=w860, bytes to read=w858, error in (no error)=w859) -> (connection ID out=w854:refnum<k5>, data out=w841:string, error out=w855:errorcluster)  [unwired: 2 in]
                n283 = TCP Read(connection ID=w854, bytes to read=2 ("读取的字节"), error in (no error)=w855) -> (connection ID out=w847:refnum<k5>, error out=w846:errorcluster)  [unwired: 2 in, 1 out]
                n284 = case shown="1" w848 {
                  tunnel: w847 -> [w890 w933]
                  tunnel: w846 -> [w889 w932]
                  tunnel: [w891 w934] -> w845
                  tunnel: [w892 w935] -> w844
                  tunnel: w842 -> [w887 w930]
                  tunnel: w841 -> [w886 w929]
                  tunnel: w838 -> [w874 w921]
                  frame 0, Default {
                    n285 = Build Path(base path=w874, name or relative path="Thumbnail" ("名称或相对路径")) -> (appended path=w876:path)
                    n286 = Build Path(base path=w874, name or relative path="Album" ("名称或相对路径")) -> (appended path=w875:path)
                    n287 = Build Path(base path=w876, name or relative path=w887) -> (appended path=w884:path)
                    n288 = Build Path(base path=w875, name or relative path=w887) -> (appended path=w882:path)
                    n289 = Build Path(base path=w884, name or relative path=w886) -> (appended path=w883:path)
                    n290 = Build Path(base path=w882, name or relative path=w886) -> (appended path=w881:path)
                    n291 = Equal?(x=w886, y="") -> (x = y?=w885:bool)
                    n292 = case shown="真" w885 {
                      tunnel: w884 -> [_ w920]
                      tunnel: w883 -> [w913 _]
                      tunnel: w882 -> [_ w919]
                      tunnel: w881 -> [w912 _]
                      tunnel: [w909 w914] -> w880
                      frame False {
                        n293 = Delete(path (use dialog)=w913) -> (error out=w911:errorcluster)  [unwired: 4 in, 2 out]
                        n294 = Delete(path (use dialog)=w912) -> (error out=w910:errorcluster)  [unwired: 4 in, 2 out]
                        n295 = Merge Errors(w911, w910) -> (w909:errorcluster)
                      }
                      frame True {
                        n296 = Delete(path (use dialog)=w920, entire hierarchy (F)=TRUE ("整个层次结构(F)")) -> (error out=w916:errorcluster)  [unwired: 3 in, 2 out]
                        n297 = Delete(path (use dialog)=w919, entire hierarchy (F)=TRUE ("整个层次结构(F)")) -> (error out=w915:errorcluster)  [unwired: 3 in, 2 out]
                        n298 = Merge Errors(w916, w915) -> (w914:errorcluster)
                      }
                    }
                    n299 = case shown="无错误" w880 {
                      tunnel: [w893 w901] -> w879
                      frame No Error {
                        n300 = Build Array(u8 85, u8 170, u8 8, u8 1 ("元素"), u8 0, u8 0) -> (w900:u8[])
                        n301 = Byte Array To String(unsigned byte array=w900) -> (string=w893:string)
                      }
                      frame Error {
                        n302 = Build Array(u8 85, u8 170, u8 8, u8 0 ("元素"), u8 0, u8 0) -> (w908:u8[])
                        n303 = Byte Array To String(unsigned byte array=w908) -> (string=w901:string)
                      }
                    }
                    n304 = TCP Write(connection ID=w890, data in=w879, error in (no error)=w889) -> (connection ID out=w891:refnum<k5>, error out=w892:errorcluster)  [unwired: 1 in, 1 out]
                  }
                  frame 1 {
                    n305 = Build Path(base path=w921, name or relative path="Music" ("名称或相对路径")) -> (appended path=w922:path)
                    n306 = Build Path(base path=w922, name or relative path=w930) -> (appended path=w927:path)
                    n307 = Build Path(base path=w927, name or relative path=w929) -> (appended path=w926:path)
                    n308 = Equal?(x=w929, y="") -> (x = y?=w928:bool)
                    n309 = case shown="真" w928 {
                      tunnel: w927 -> [_ w956]
                      tunnel: w926 -> [w953 _]
                      tunnel: [w952 w954] -> w925
                      frame False {
                        n310 = Delete(path (use dialog)=w953) -> (error out=w952:errorcluster)  [unwired: 4 in, 2 out]
                      }
                      frame True {
                        n311 = Delete(path (use dialog)=w956, entire hierarchy (F)=TRUE ("整个层次结构(F)")) -> (error out=w954:errorcluster)  [unwired: 3 in, 2 out]
                      }
                    }
                    n312 = case shown="无错误" w925 {
                      tunnel: [w936 w944] -> w924
                      frame No Error {
                        n313 = Build Array(u8 85, u8 170, u8 8, u8 1 ("元素"), u8 0, u8 0) -> (w943:u8[])
                        n314 = Byte Array To String(unsigned byte array=w943) -> (string=w936:string)
                      }
                      frame Error {
                        n315 = Build Array(u8 85, u8 170, u8 8, u8 0 ("元素"), u8 0, u8 0) -> (w951:u8[])
                        n316 = Byte Array To String(unsigned byte array=w951) -> (string=w944:string)
                      }
                    }
                    n317 = TCP Write(connection ID=w933, data in=w924, error in (no error)=w932) -> (connection ID out=w934:refnum<k5>, error out=w935:errorcluster)  [unwired: 1 in, 1 out]
                  }
                }
              }
              frame 9 {
                n318 = TCP Read(connection ID=w970, bytes to read=4 ("读取的字节"), error in (no error)=w969) -> (connection ID out=w983:refnum<k5>, error out=w981:errorcluster)  [unwired: 2 in, 1 out]
                n319 = TCP Read(connection ID=w983, bytes to read=1 ("读取的字节"), error in (no error)=w981) -> (connection ID out=w978:refnum<k5>, data out=w979:string, error out=w977:errorcluster)  [unwired: 2 in]
                n320 = Type Cast(type=w968, x=w979) -> (*(type *) &x=w967:u8)
                n321 = TCP Read(connection ID=w978, bytes to read=1 ("读取的字节"), error in (no error)=w977) -> (connection ID out=w975:refnum<k5>, data out=w971:string, error out=w974:errorcluster)  [unwired: 2 in]
                n322 = Type Cast(type=w968, x=w971) -> (*(type *) &x=w973:u8)
                n323 = Current VI's Path() -> (path=w961:path)
                n324 = Strip Path(path=w961) -> (stripped path=w960:path)  [unwired: 1 out]
                n325 = TCP Read(connection ID=w975, bytes to read=w973, error in (no error)=w974) -> (connection ID out=w958:refnum<k5>, data out=w962:string, error out=w959:errorcluster)  [unwired: 2 in]
                n326 = Strip Path(path=w960) -> (stripped path=w957:path)  [unwired: 1 out]
                n327 = TCP Read(connection ID=w958, bytes to read=2 ("读取的字节"), error in (no error)=w959) -> (connection ID out=w966:refnum<k5>, error out=w965:errorcluster)  [unwired: 2 in, 1 out]
                n328 = case shown="0, 默认" w967 {
                  tunnel: w966 -> [w998 w1025]
                  tunnel: w965 -> [w997 w1024]
                  tunnel: [w999 w1026] -> w964
                  tunnel: [w1000 w1027] -> w963
                  tunnel: w962 -> [w996 w1023]
                  tunnel: w957 -> [w987 w1019]
                  frame 0, Default {
                    n329 = Build Path(base path=w987, name or relative path="Thumbnail" ("名称或相对路径")) -> (appended path=w986:path)
                    n330 = Build Path(base path=w987, name or relative path="Album" ("名称或相对路径")) -> (appended path=w985:path)
                    n331 = Build Path(base path=w986, name or relative path=w996) -> (appended path=w995:path)
                    n332 = Build Path(base path=w985, name or relative path=w996) -> (appended path=w994:path)
                    n333 = Create Folder(path (use dialog)=w995) -> (error out=w991:errorcluster)  [unwired: 2 in, 2 out]
                    n334 = Create Folder(path (use dialog)=w994) -> (error out=w990:errorcluster)  [unwired: 2 in, 2 out]
                    n335 = Merge Errors(w991, w990) -> (w993:errorcluster)
                    n336 = case shown="无错误" w993 {
                      tunnel: [w1001 w1009] -> w992
                      frame No Error {
                        n337 = Build Array(u8 85, u8 170, u8 9, u8 1 ("元素"), u8 0, u8 0) -> (w1008:u8[])
                        n338 = Byte Array To String(unsigned byte array=w1008) -> (string=w1001:string)
                      }
                      frame Error {
                        n339 = Build Array(u8 85, u8 170, u8 9, u8 0 ("元素"), u8 0, u8 0) -> (w1016:u8[])
                        n340 = Byte Array To String(unsigned byte array=w1016) -> (string=w1009:string)
                      }
                    }
                    n341 = TCP Write(connection ID=w998, data in=w992, error in (no error)=w997) -> (connection ID out=w999:refnum<k5>, error out=w1000:errorcluster)  [unwired: 1 in, 1 out]
                  }
                  frame 1 {
                    n342 = Build Path(base path=w1019, name or relative path="Music" ("名称或相对路径")) -> (appended path=w1018:path)
                    n343 = Build Path(base path=w1018, name or relative path=w1023) -> (appended path=w1022:path)
                    n344 = Create Folder(path (use dialog)=w1022) -> (error out=w1017:errorcluster)  [unwired: 2 in, 2 out]
                    n345 = case shown="无错误" w1017 {
                      tunnel: [w1028 w1036] -> w1021
                      frame No Error {
                        n346 = Build Array(u8 85, u8 170, u8 9, u8 1 ("元素"), u8 0, u8 0) -> (w1035:u8[])
                        n347 = Byte Array To String(unsigned byte array=w1035) -> (string=w1028:string)
                      }
                      frame Error {
                        n348 = Build Array(u8 85, u8 170, u8 9, u8 0 ("元素"), u8 0, u8 0) -> (w1043:u8[])
                        n349 = Byte Array To String(unsigned byte array=w1043) -> (string=w1036:string)
                      }
                    }
                    n350 = TCP Write(connection ID=w1025, data in=w1021, error in (no error)=w1024) -> (connection ID out=w1026:refnum<k5>, error out=w1027:errorcluster)  [unwired: 1 in, 1 out]
                  }
                }
              }
            }
          }
        }
      }
    }
  }
  "error out" <- w2
  "IP 2" <- w3
  "exit" <- w1
